vi "Get Point Data Map.vi"(11 "Task Actor in":refnum<class "Task Actor.lvclass">) -> (2 "Data Map":map{string, variant}(c390), 3 "Task Actor out":refnum<class "Task Actor.lvclass">)   [LabVIEW 2024, in "Task Actor.lvlib" / "Task Actor.lvclass"]
uses:
  Task Actor.lvclass
  Task Actor.lvclass/Task Actor.ctl
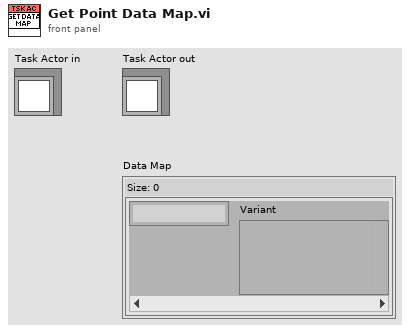
[diagram p1: front panel]
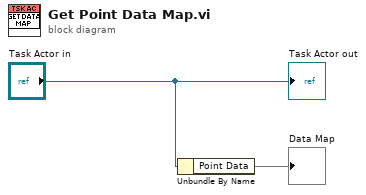
[diagram p0: block diagram]
diagram:
  n1 = Unbundle By Name("Task Actor in") -> ("Point Data"=→"Data Map":map{string, variant})
  "Task Actor out" <- "Task Actor in"
